vi "Blink 3 simple and correct one.vi"(8 "Error In":errorcluster, 10 "numberInput1":dbl) -> (0 "Error Out":errorcluster, 3 "BoolArrayIndicator1":bool[](array[boolean]))   [LabVIEW 2014]
uses:
  UserDefined StructType.ctl
  UserDefined StructType 2.ctl
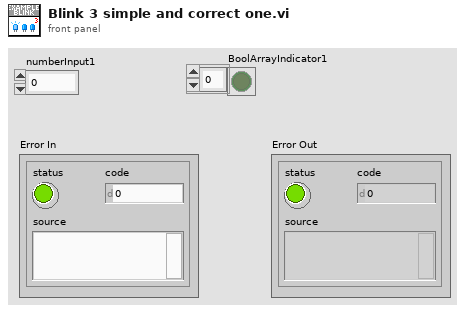
[diagram p1: front panel]
types:
  T1 = typedef "UserDefined StructType 2.ctl" = cluster{"cisloA":i32, "cisloB":u8}
  T2 = typedef "UserDefined StructType.ctl" = cluster{"LuboString":string, "NumInsideUserCluter":i32, "Double insideCluster":dbl}
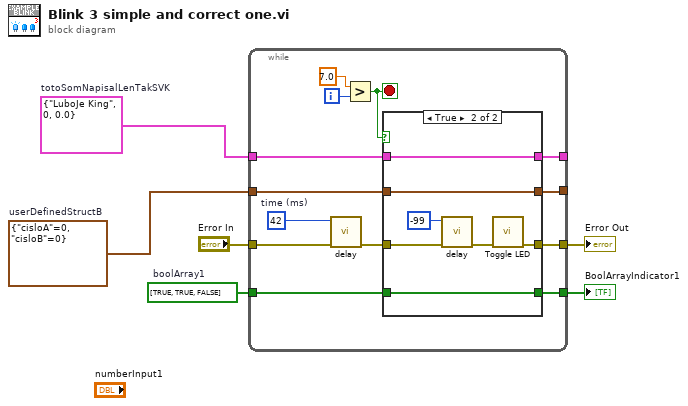
[diagram p0: block diagram]
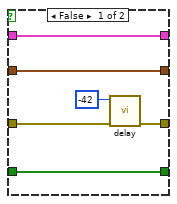
[diagram p2: hidden frame]
diagram:
  w1 = T1 {"cisloA"=0, "cisloB"=0}  # userDefinedStructB
  w2 = T2 {"LuboString"="LuboJe King", "NumInsideUserCluter"=0, "Double insideCluster"=0.0}  # totoSomNapisalLenTakSVK
  w4 = bool[] [TRUE, TRUE, FALSE]  # boolArray1
  n1 = while {
    tunnel: "Error In" -> [w19]
    tunnel: [w14] -> w5
    tunnel: w4 -> [w11]
    tunnel: [w12] -> w3
    tunnel: w2 -> [w9]
    tunnel: [w10] -> _
    tunnel: [w8] -> _
    tunnel: w1 -> [w7]
    i -> [w17]
    stop <- w13 stop-if-true
    w15 = 42  # time (ms)
    n2 = call "delay.vi"("Error In"=w19, "time (ms)"=w15) -> ("Error Out"=w18:errorcluster)  [unwired: 9 in]
    n3 = Greater?(x=7.0, y=w17) -> (0:w13:bool)
    n4 = case shown="True" w13 {
      tunnel: w18 -> [w25 w31]
      tunnel: [w24 w32] -> w14
      tunnel: [w22 w28] -> w12
      tunnel: w11 -> [w22 w28]
      tunnel: [w21 w27] -> w10
      tunnel: w9 -> [w21 w27]
      tunnel: [w20 w26] -> w8
      tunnel: w7 -> [w20 w26]
      frame False {
        n5 = call "delay.vi"("Error In"=w25, "time (ms)"=-42) -> ("Error Out"=w24:errorcluster)  [unwired: 9 in]
      }
      frame True {
        n6 = call "delay.vi"("Error In"=w31, "time (ms)"=-99) -> ("Error Out"=w30:errorcluster)  [unwired: 9 in]
        n7 = call "Toggle LED.vi"("Error In"=w30) -> ("Error Out"=w32:errorcluster)  [unwired: 10 in]
      }
    }
  }
  "Error Out" <- w5
  "BoolArrayIndicator1" <- w3
